vi "Get  PreCurrentTime.vi"(0 "hour":i32, 11 "error in (no error)":errorcluster) -> (4 "current time":timestamp, 6 "CurrStr":string, 8 "Pretime stamp":timestamp, 10 "PreStr":string, 15 "error out":errorcluster)   [LabVIEW 2014]
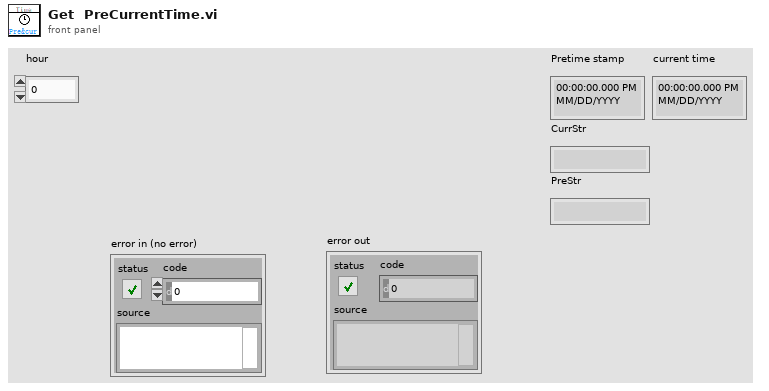
[diagram p1: front panel]
types:
  T1 = typedef "LVDateTimeRec.ctl" = cluster{"fractional second":dbl, "second":i32, "minute":i32, "hour":i32, "day of month":i32, "month":i32, "year":i32, "day of week":i32, "day of year":i32, "DST":i32}
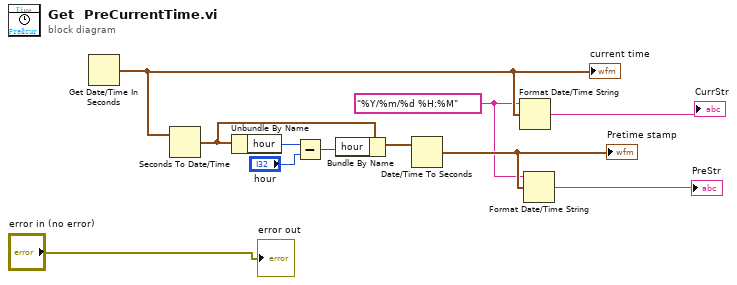
[diagram p0: block diagram]
diagram:
  w3 = "%Y/%m/%d %H:%M"
  n1 = Get Date/Time In Seconds() -> (seconds since 1Jan1904=w6:timestamp)
  "current time" <- w6
  n2 = Seconds To Date/Time(time stamp (now)=w6) -> (date time rec=w11:T1)  [unwired: 1 in]
  n3 = Unbundle By Name(w11) -> ("hour"=w10:i32)
  n4 = Subtract(x=w10, y="hour") -> (x-y=w9:i32)
  n5 = Bundle By Name(cluster=w11, "hour"=w9) -> (w7:T1)
  n6 = Date/Time To Seconds(2:w7) -> (0:w4:timestamp)  [unwired: 1 in]
  "Pretime stamp" <- w4
  n7 = Format Date/Time String(time format string (%c)=w3, seconds (now)=w6) -> (date/time string=→"CurrStr":string)  [unwired: 1 in]
  n8 = Format Date/Time String(time format string (%c)=w3, seconds (now)=w4) -> (date/time string=→"PreStr":string)  [unwired: 1 in]
  "error out" <- "error in (no error)"
